vi "new resize Tbl 1D.vi"(9 "Bounds":T4, 10 "Display Cluster In":T1={"Initialization"=TRUE, "Show In and out values"=TRUE, "Show Highliting"=TRUE, "Open Plot"=FALSE, "Format String"="%10_4g", "Limits"={"Min X"=-inf, "Max X"=inf, "MaxDiff X"=inf, "MaxGrad X"=inf, "Min Y"=-inf, "Max Y"=inf, "MaxDiff Y"=inf}, "Vertical Scrollbar"=FALSE, "Data"={"X"=[0.0, 5.0], "Y"=[0.0, 100.0]}, "Undo Avaliable"=FALSE, "NIVS.System Definition Root"=refnum, "Selected Parameter"="", "Selected Working Pt"=0.0, "X"=0.0} caption="State", 11 "1D Table":refnum<vi>) -> ()   [LabVIEW 2011, in "TBL1D.xctl"]
uses:
  TBL1D.xctl
  <vilib>/Utility/miscctls.llb/LVRectTypeDef.ctl
  State TBL1D.ctl
  Limits TBL1D.ctl
  Data TBL1D.ctl
  NationalInstruments.VeriStand.SystemStorage
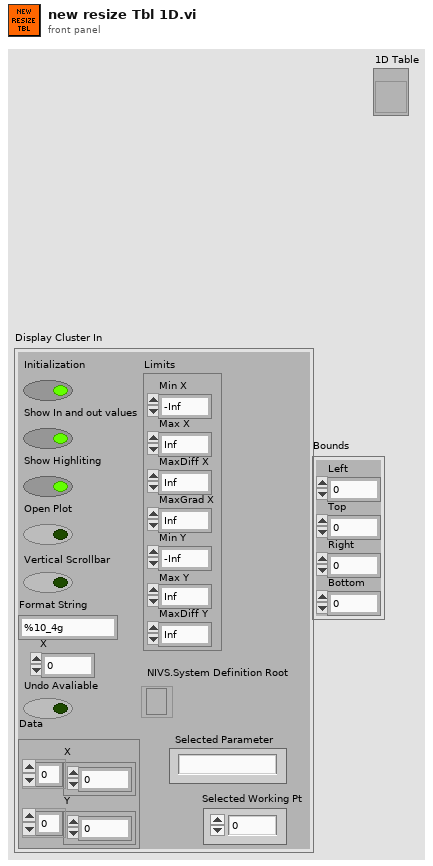
[diagram p1: front panel]
types:
  T1 = typedef "TBL1D.xctl/State TBL1D.ctl" = cluster{"Initialization":bool, "Show In and out values":bool, "Show Highliting":bool, "Open Plot":bool, "Format String":string, "Limits":T2, "Vertical Scrollbar":bool, "Data":T3, "Undo Avaliable":bool, "NIVS.System Definition Root":refnum<k24>, "Selected Parameter":string, "Selected Working Pt":dbl, "X":sgl}
  T2 = typedef "TBL1D.xctl/Limits TBL1D.ctl" = cluster{"Min X":sgl, "Max X":sgl, "MaxDiff X":sgl, "MaxGrad X":sgl, "Min Y":sgl, "Max Y":sgl, "MaxDiff Y":sgl}
  T3 = typedef "TBL1D.xctl/Data TBL1D.ctl" = cluster{"X":sgl[], "Y":sgl[]}
  T4 = typedef "LVRectTypeDef.ctl" = cluster{"Left":i16, "Top":i16, "Right":i16, "Bottom":i16}
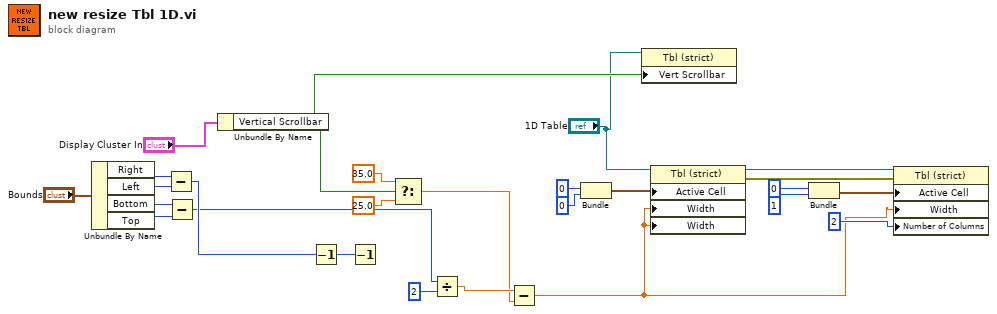
[diagram p0: block diagram]
diagram:
  n1 = Unbundle By Name("Bounds") -> ("Right"=w15:i16, "Left"=w14:i16, "Bottom"=w13:i16, "Top"=w12:i16)
  n2 = Subtract(x=w15, y=w14) -> (x-y=w9:i16)
  n3 = Subtract(x=w13, y=w12) -> (x-y=w6:i16)
  n4 = Unbundle By Name("Display Cluster In") -> ("Vertical Scrollbar"=w7:bool)
  n5 = Decrement(x=w9) -> (x-1=w8:i16)
  n6 = Decrement(x=w8) -> ()  [unwired: 1 out]
  n7 = Select(t=35.0 ("y"), s=w7, f=25.0 ("y")) -> (s? t:f=w3:dbl)
  n8 = Divide(x=w6, y=i16 2) -> (x/y=w4:dbl)
  n9 = Subtract(x=w4, y=w3) -> (x-y=w1:dbl)
  n10 = Bundle("y"=i16 0, "y"=i16 0) -> (w24:cluster{"y":i16, "y":i16})  [unwired: 1 out]
  n11 = property on="Property Node" class="Tbl (strict)"(reference="1D Table", "Vert Scrollbar"=w7) -> ()  [unwired: 1 in, 2 out]
  n12 = property on="Property Node" class="Tbl (strict)"(reference="1D Table", "Active Cell"=w24, "Width"=w1, "Width"=w1) -> (reference out=w18:refnum<vi>, error out=w19:errorcluster)  [unwired: 1 in]
  n13 = Bundle("y"=i16 0, "y"=i16 1) -> (w21:cluster{"y":i16, "y":i16})  [unwired: 1 out]
  n14 = property on="Property Node" class="Tbl (strict)"(reference=w18, error in=w19, "Active Cell"=w21, "Width"=w1, "Number of Columns"=u32 2 ("Number of Rows")) -> ()  [unwired: 2 out]
